vi "State Logic.vi"(0 "TLB' data in":refnum<class "Springboard TLB`.lvclass">, 1 "process state logic enable":bool, 5 "trigger queue in":refnum<queue>, 7 "action queue in":refnum<queue>, 11 "error in":errorcluster) -> (4 "TLB' data out":refnum<class "Springboard TLB`.lvclass">, 15 "error out":errorcluster)   [LabVIEW 2018, in "Springboard TLB`.lvlib" / "Springboard TLB`.lvclass"]
doc: "Control process for TLB' template.\n\n<B>Input Parameters</B>\n\n<B>TLB' data in</B> is the templates' private data.\n\n<B>process state logic enable</B> enable state logic change.\n\n<B>trigger queue in</B> is a reference to a queue. Use the Create Trigger Queue function to obtain a queue reference. \n\n<B>action queue in</B> is a reference to a queue. Use the Create Action Queue function to obtain a queue reference. \n\n<B>timeout (ms)</B> queue timeout.\n\n<B>error in</B> describes error conditions that occur before this node runs. This input provides standard error in functionality.\n\n<B>Output Parameters</B>\n\n<B>TLB' data out</B> is the templates' private data.\n\n<B>error out</B> contains error information. This output provides standard error out functionality."
uses:
  Springboard TLB`.lvclass
  Application Components/Trigger API/System Trigger Element.ctl
  Application Components/Trigger API/System Trigger.ctl
  Core Components/Actions/System Action Element.ctl
  Springboard TLB`.lvclass/Springboard TLB`.ctl
  State.ctl
  Core Components/Error Handler/TLB` Error Handler.lvclass/TLB` Error Handler.ctl
  Core Components/Error Handler/accessors/Get Action Causing Error.vi
  Core Components/Error Handler/accessors/Get Originating State.vi
  Core Components/Error Handler/accessors/Get Destination State.vi
  Core Components/Error Handler/accessors/Get Executed System Actions.vi
  Core Components/Error Handler/accessors/Get Remaing System Actions.vi
  Core Components/Error Handler/Core/actions/support/Error FLUSH-LOG-DIALOG.vi
  Core Components/Error Handler/Core/actions/support/Error FLUSH-DIALOG.vi
  Application Components/Configuration/Springboard Station Configuration.lvclass
  Application Components/Trigger API/Springboard Trigger API.lvlib
  Core Components/Error Handler/TLB` Error Handler.lvclass
  Core Components/Actions/Actions.lvlib
  Springboard TLB`.lvlib
  <vilib>/Utility/config.llb/NI_LVConfig.lvlib
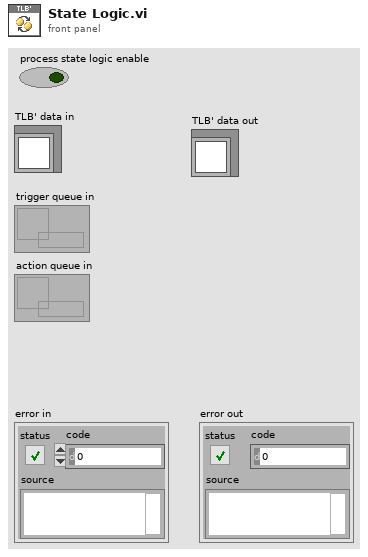
[diagram p1: front panel]
types:
  T1 = typedef "Springboard TLB`.lvlib/Springboard TLB`.lvclass/State.ctl" = enum16{"<Startup>", "Idle", "Evaluate Build Directory", "Creating", "Evaluate Build", "<Shutdown>", "<Error>"}
  T2 = typedef "Springboard TLB`.lvlib/Springboard Trigger API.lvlib/System Trigger.ctl" = enum16{"<None>", "<Return to Safe State Actions>", "<Cache User Parameters>", "<Close Application>", "<Error>", "Create New", "Abort Creation", "Cancel"}
  T3 = typedef "NI_LVConfig.lvlib/Config Data RefNum.ctl" = refnum<k1>
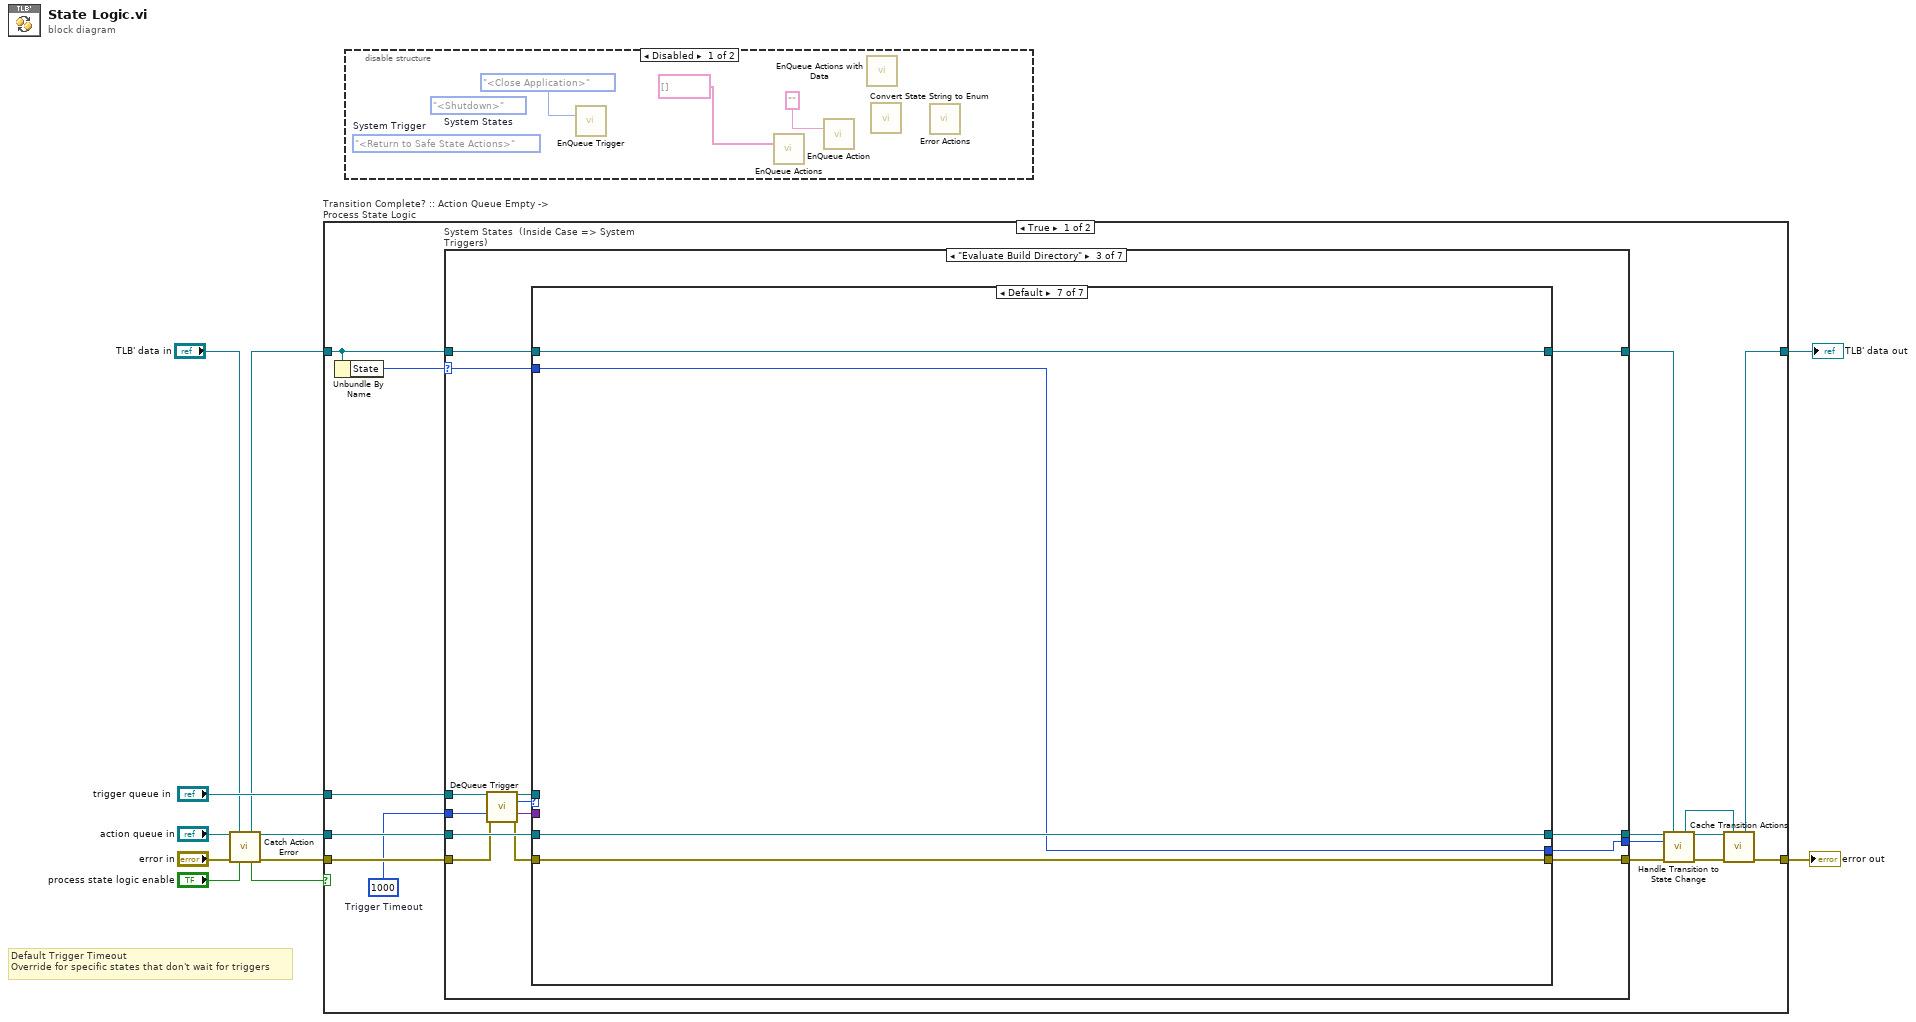
[diagram p0: block diagram]
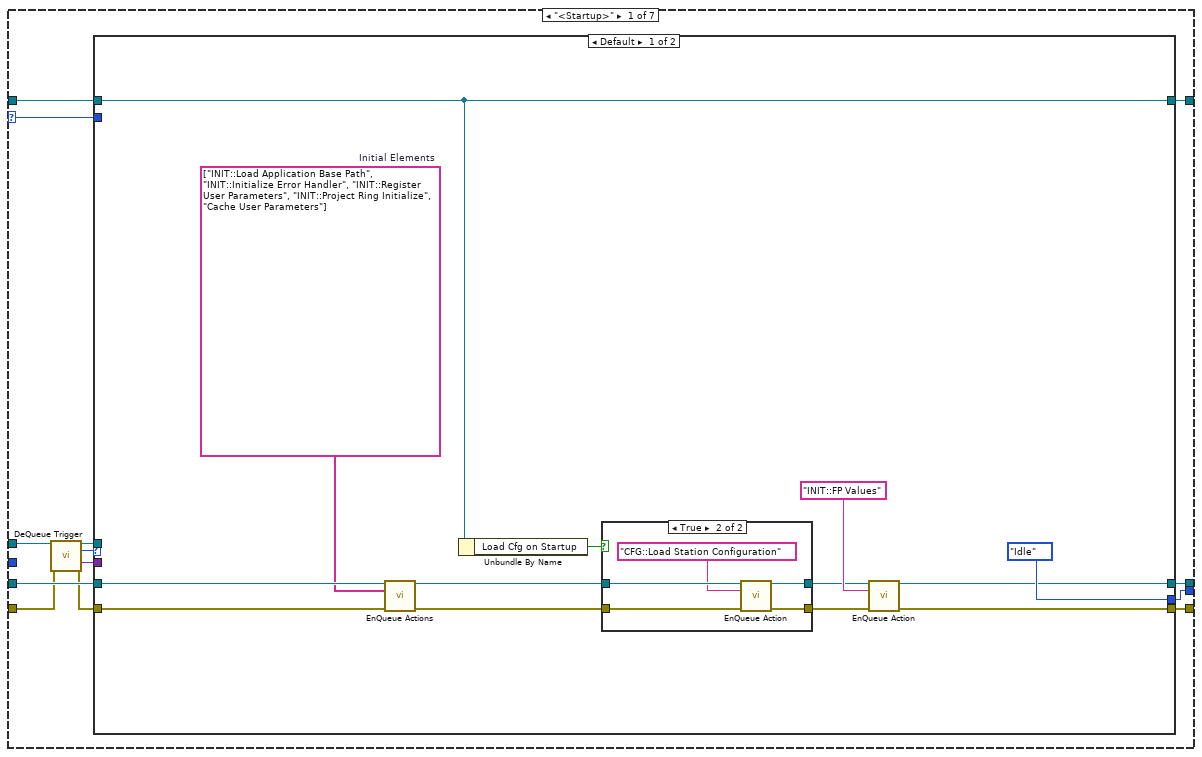
[diagram p3: hidden frame]
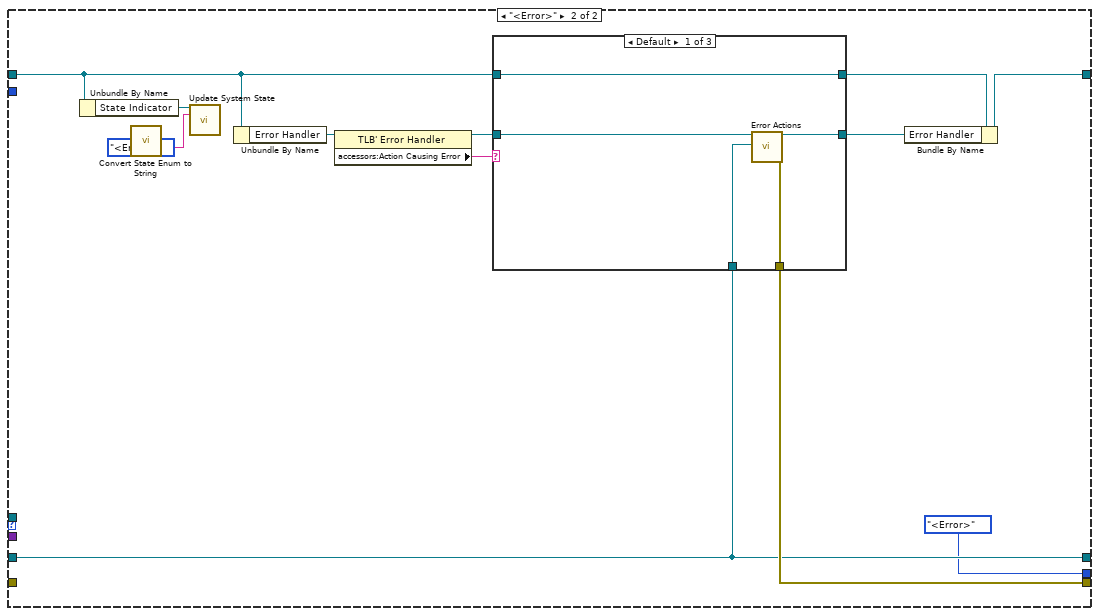
[diagram p5: hidden frame]
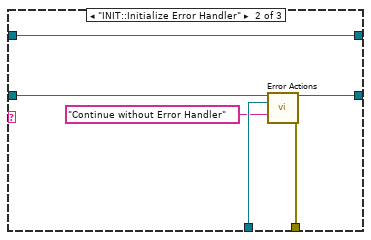
[diagram p6: hidden frame]
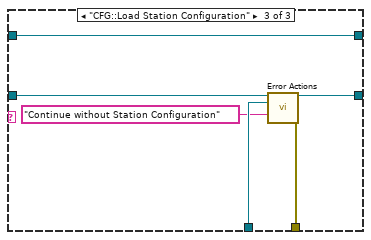
[diagram p7: hidden frame]
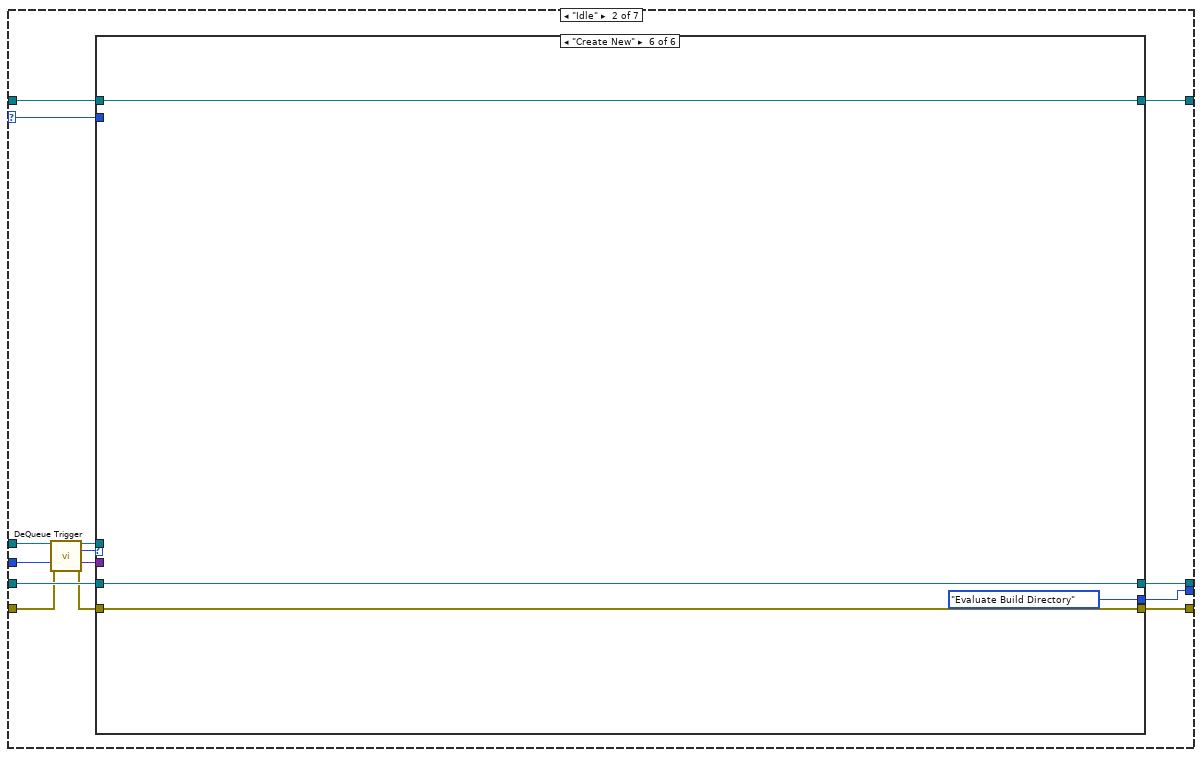
[diagram p8: hidden frame]
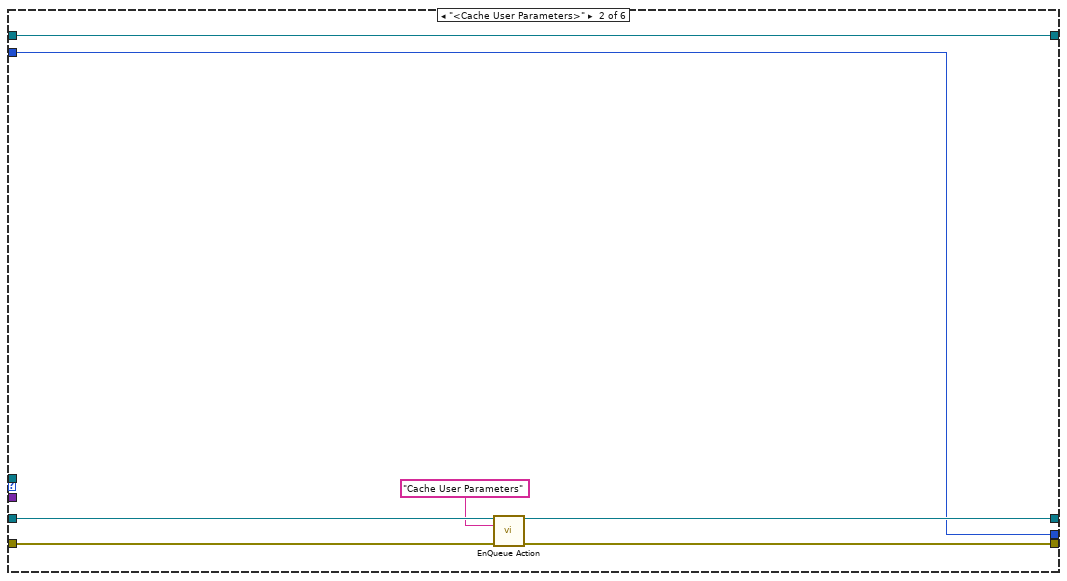
[diagram p10: hidden frame]
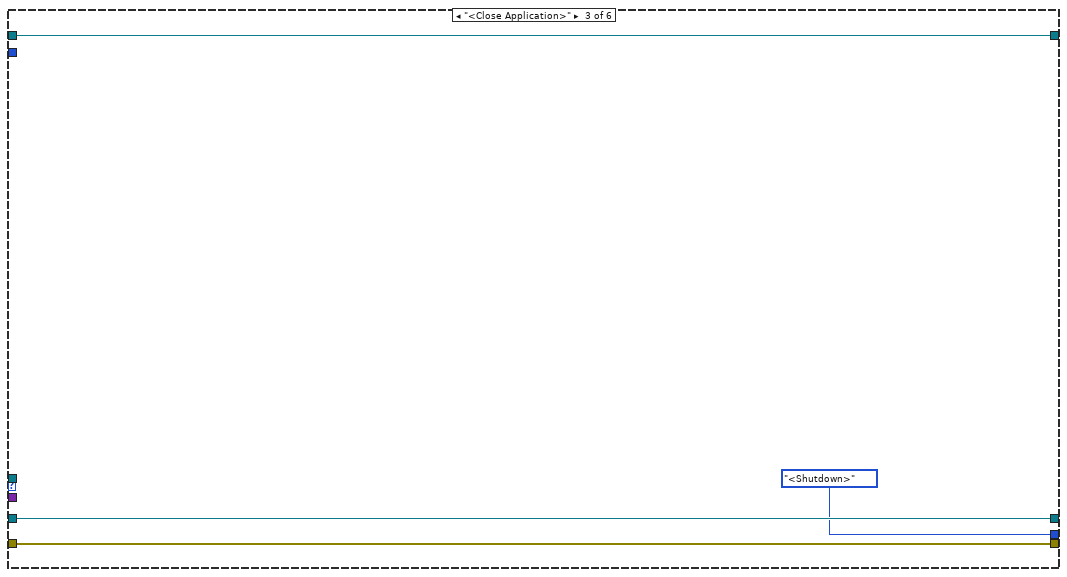
[diagram p11: hidden frame]
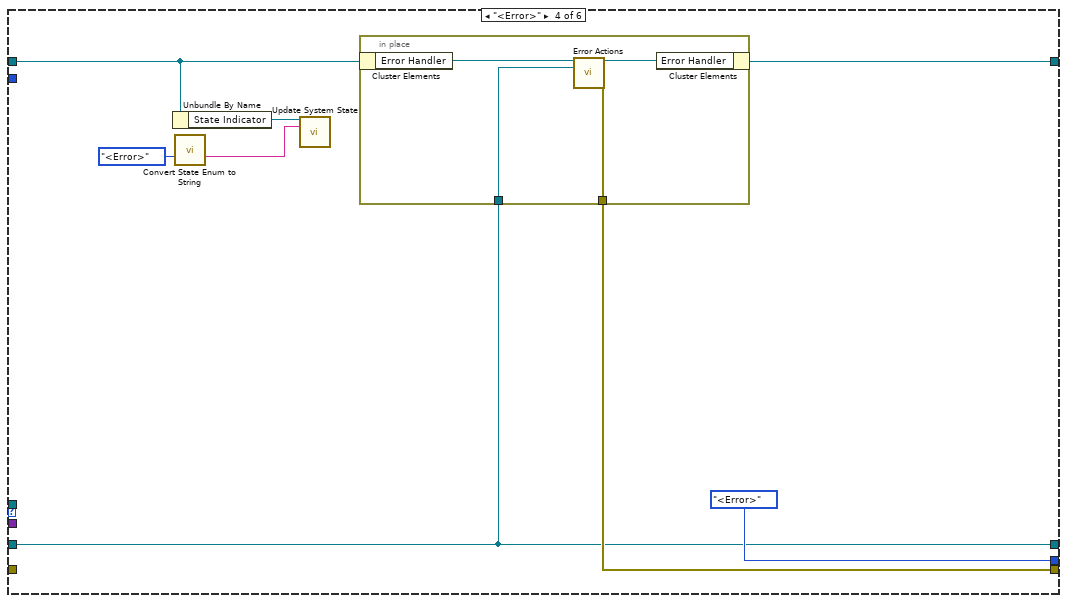
[diagram p12: hidden frame]
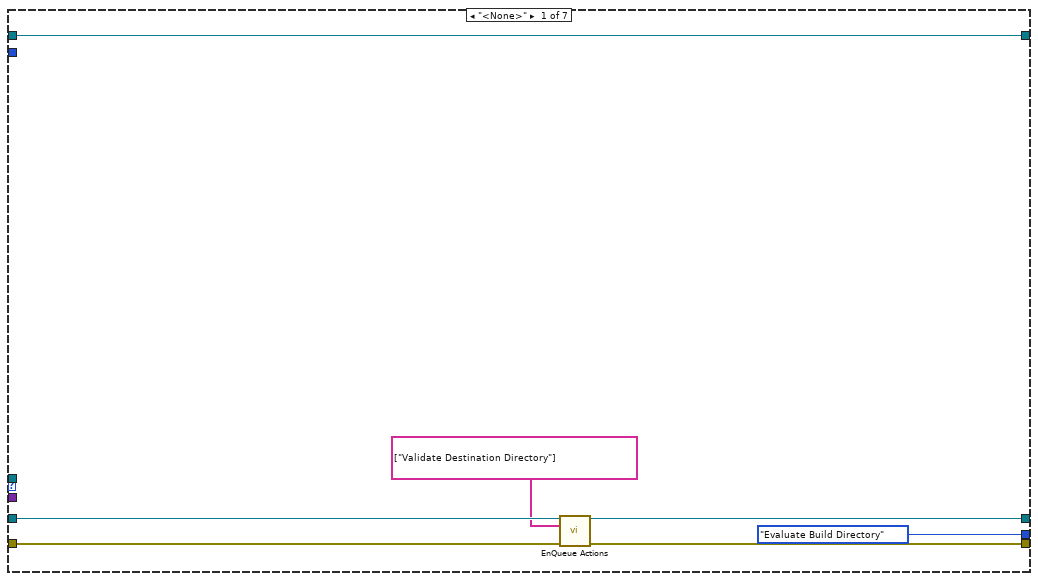
[diagram p14: hidden frame]
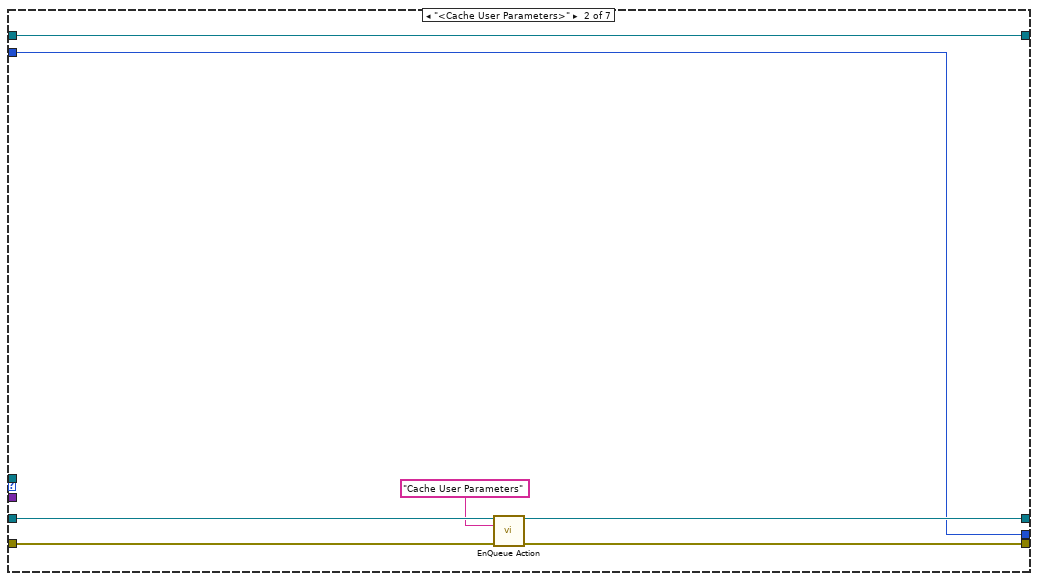
[diagram p15: hidden frame]
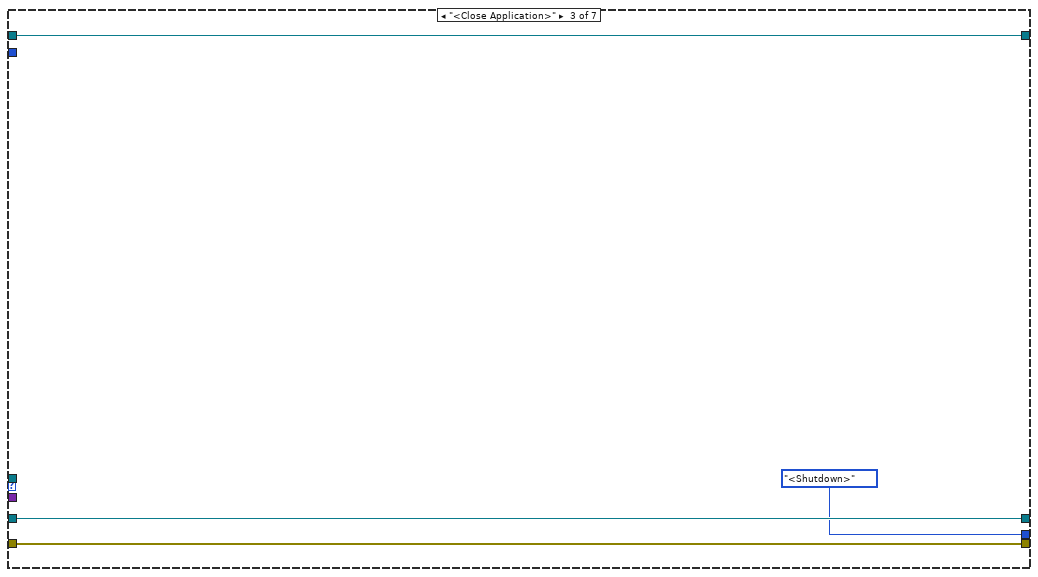
[diagram p16: hidden frame]
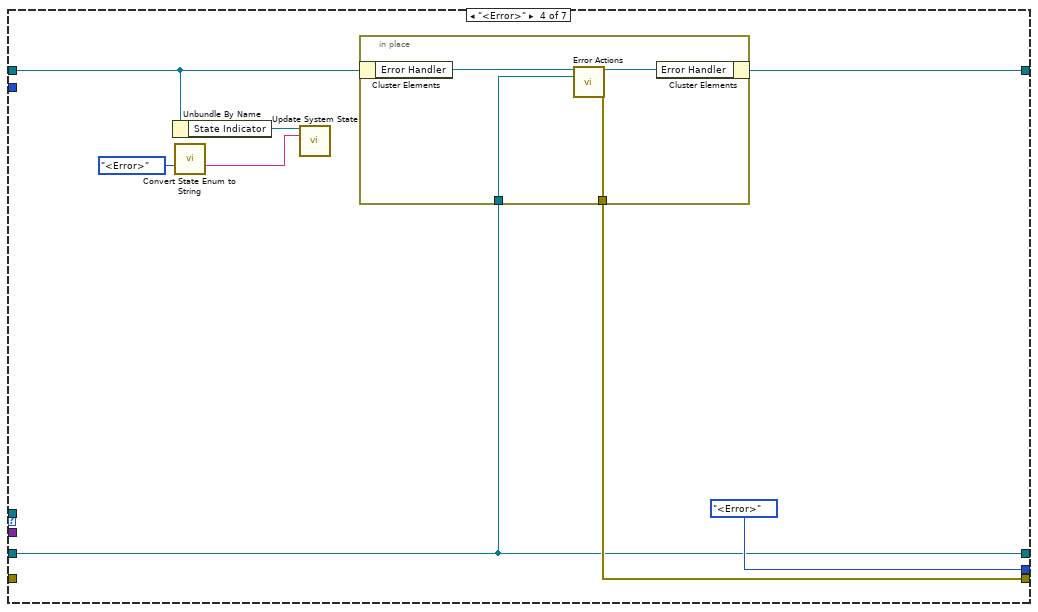
[diagram p17: hidden frame]
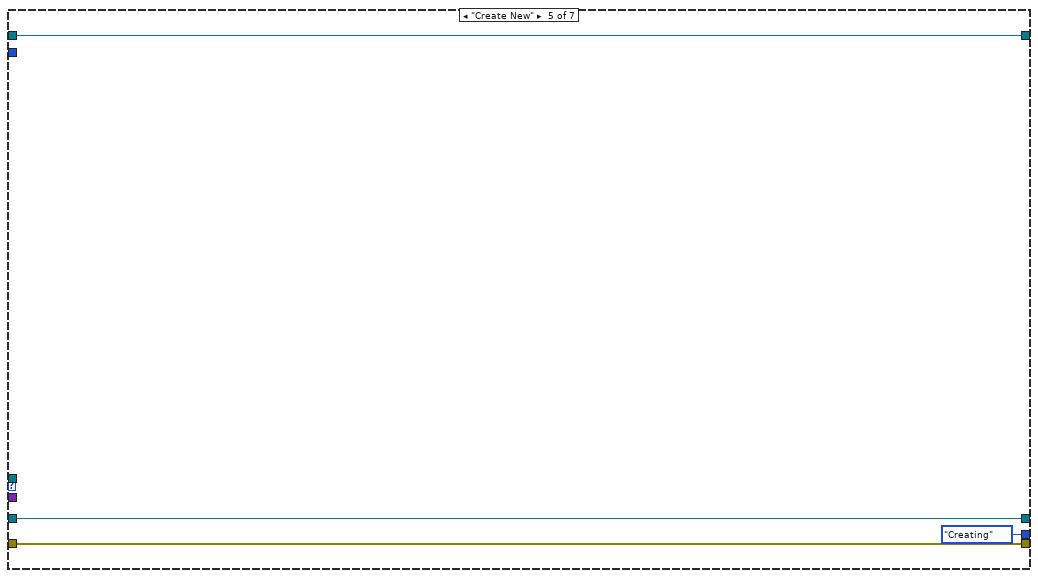
[diagram p18: hidden frame]
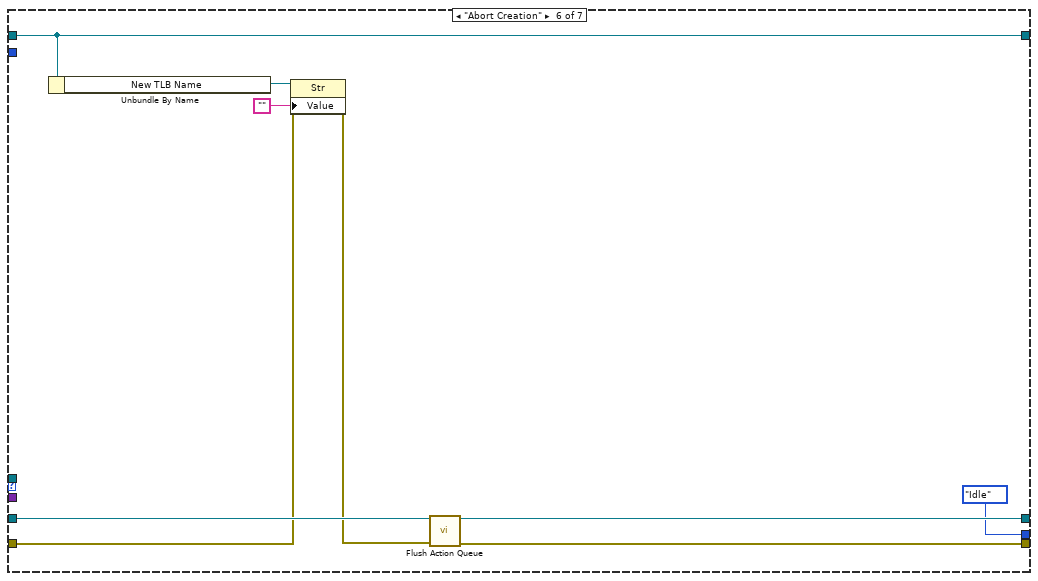
[diagram p19: hidden frame]
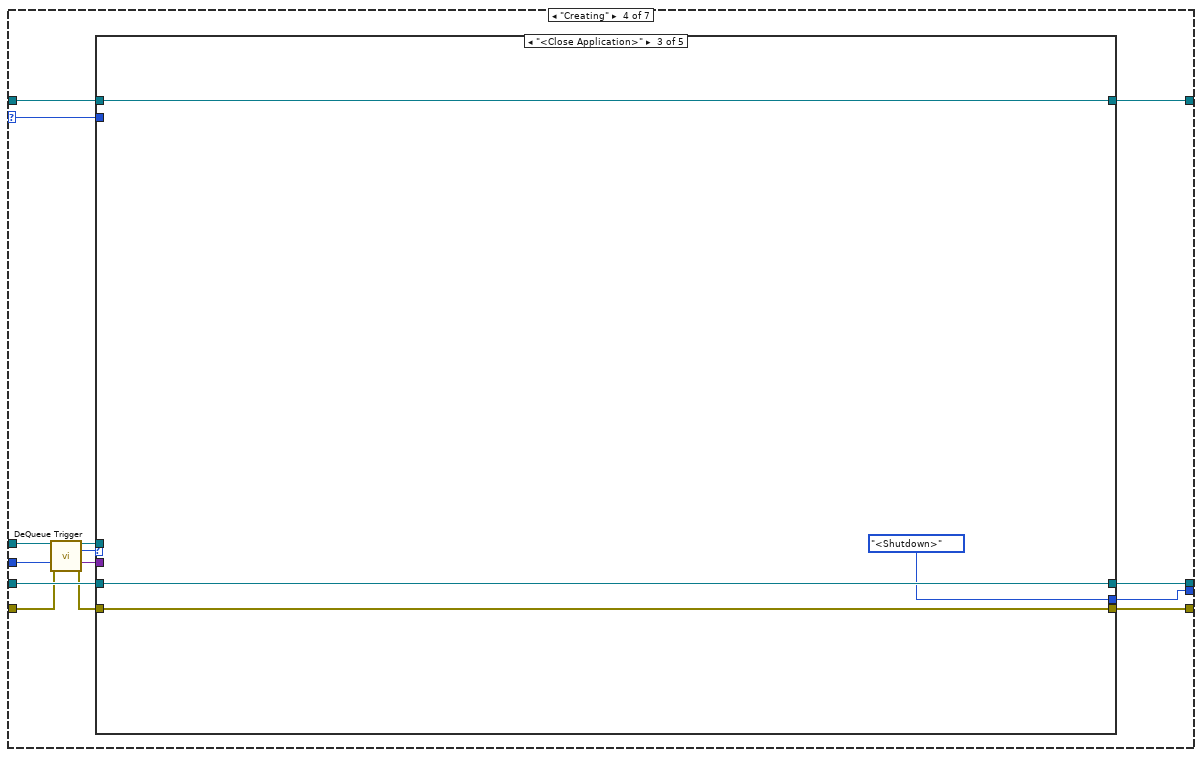
[diagram p20: hidden frame]
diagram:
  # "Default Trigger Timeout\nOverride for specific states that don't wait for triggers"
  n1 = call "Catch Action Error.vi"("action queue in"="action queue in", "TLB' Template in"="TLB' data in", "error in (no error)"="error in", "process state logic enable in"="process state logic enable") -> ("TLB' Template out"=w6:refnum<class "Springboard TLB`.lvclass">, "action queue in"=w2:refnum<queue>, "process state logic enable out"=w4:bool, "error out"=w7:errorcluster)  [unwired: 8 in]
  n2 = case "Transition Complete? :: Action Queue Empty -> Process State Logic" shown="True" w4 {
    tunnel: [w17 w559] -> w10
    tunnel: w6 -> [w22 w559]
    tunnel: w7 -> [w26 w560]
    tunnel: w2 -> [w25 _]
    tunnel: [w20 w560] -> w11
    tunnel: "trigger queue in" -> [w24 _]
    frame True {
      w18 = 1000  # Trigger Timeout
      n3 = Unbundle By Name(w22) -> ("State"=w19:T1)
      n4 = case "System States  (Inside Case => System Triggers)" shown="\"Evaluate Build Directory\"" w19 {
        selector: w19 -> [w27 w92 w141 w202 w250 w324 _]
        tunnel: [w33 w97 w146 w207 w255 w322 w557] -> w15
        tunnel: w22 -> [w34 w98 w147 w208 w256 w323 w557]
        tunnel: w26 -> [w32 w96 w145 w206 w254 w321 w556]
        tunnel: w25 -> [w38 w102 w151 w212 w260 w325 w555]
        tunnel: [w37 w101 w150 w211 w259 w328 w553] -> w23
        tunnel: w24 -> [w39 w103 w152 w213 w261 w329 _]
        tunnel: [w36 w100 w149 w210 w258 w327 w554] -> w16
        tunnel: [w35 w99 w148 w209 w257 w326 State."<Shutdown>" ("State")] -> w12
        tunnel: w18 -> [_ w91 w140 w201 w249 _ _]
        frame "<Startup>" {
          n5 = call "DeQueue Trigger.vi"("trigger queue in"=w39, "error in"=w32) -> ("trigger queue out"=w28:refnum<queue>, "system trigger"=w30:T2, "trigger data"=w29:variant, "error out"=w31:errorcluster)  [unwired: 10 in]
          n6 = case shown="Default" w30 {
            tunnel: w31 -> [w49 _]
            tunnel: w38 -> [w51 w70]
            tunnel: [w40 w71] -> w37
            tunnel: [w42 w70] -> w36
            tunnel: w29 -> [_ _]
            tunnel: [State."Idle" ("State") State."<Error>" ("State")] -> w35
            tunnel: w34 -> [w47 w61]
            tunnel: [w47 w72] -> w33
            tunnel: w28 -> [_ _]
            tunnel: w27 -> [_ _]
            frame Default {
              w50 = string[] ["INIT::Load Application Base Path", "INIT::Initialize Error Handler", "INIT::Register User Parameters", "INIT::Project Ring Initialize", "Cache User Parameters"]  # Initial Elements
              n7 = call "EnQueue Actions.vi"("action queue in"=w51, "actions"=w50, "error in"=w49) -> ("action queue out"=w46:refnum<queue>, "error out"=w48:errorcluster)  [unwired: 11 in]
              n8 = Unbundle By Name(w47) -> ("Load Cfg on Startup"=w45:bool)
              n9 = case shown="True" w45 {
                tunnel: w48 -> [w53 w59]
                tunnel: [w53 w58] -> w41
                tunnel: w46 -> [w54 w57]
                tunnel: [w54 w56] -> w43
                frame False {
                }
                frame True {
                  n10 = call "EnQueue Action.vi"("action queue in"=w57, "action"="CFG::Load Station Configuration", "error in"=w59) -> ("action queue out"=w56:refnum<queue>, "error out"=w58:errorcluster)  [unwired: 11 in]
                }
              }
              n11 = call "EnQueue Action.vi"("action queue in"=w43, "action"="INIT::FP Values", "error in"=w41) -> ("action queue out"=w42:refnum<queue>, "error out"=w40:errorcluster)  [unwired: 11 in]
            }
            frame "<Error>" {
              n12 = Unbundle By Name(w61) -> ("State Indicator"=w65:refnum<user-event>)
              n13 = call "Convert State Enum to String.vi"("state in"=State."<Error>") -> ("state out"=w64:string)  [unwired: 13 in, 1 out]
              n14 = call "Update System State.vi"("State Indicator"=w65, "system state message"=w64) -> ()  [unwired: 13 in, 1 out]
              n15 = Unbundle By Name(w61) -> ("Error Handler"=w67:refnum<class "TLB` Error Handler.lvclass">)
              n16 = property class="TLB' Error Handler"(reference=w67) -> (reference out=w66:refnum<class "TLB` Error Handler.lvclass">, "accessors:Action Causing Error"=w63:string)  [unwired: 1 in, 1 out]
              n17 = case shown="Default" w63 {
                tunnel: [w75 w83 w89] -> w71
                tunnel: w70 -> [w74 w82 w88]
                tunnel: [w76 w81 w87] -> w68
                tunnel: w66 -> [w77 w80 w86]
                tunnel: w61 -> [w73 w78 w84]
                tunnel: [w73 w78 w84] -> w60
                frame Default {
                  n18 = call-poly "Error Actions.vi"("Error Handler in"=w77, "action queue in"=w74) -> ("Error Handler out"=w76:refnum<class "TLB` Error Handler.lvclass">, "error out"=w75:errorcluster)  [unwired: 12 in]
                }
                frame "INIT::Initialize Error Handler" {
                  n19 = call-poly "Error Actions.vi"("Error Handler in"=w80, "action queue in"=w82, "error button text (Return to Safe State)"="Continue without Error Handler") -> ("Error Handler out"=w81:refnum<class "TLB` Error Handler.lvclass">, "error out"=w83:errorcluster)  [unwired: 11 in]
                }
                frame "CFG::Load Station Configuration" {
                  n20 = call-poly "Error Actions.vi"("Error Handler in"=w86, "action queue in"=w88, "error button text (Return to Safe State)"="Continue without Station Configuration") -> ("Error Handler out"=w87:refnum<class "TLB` Error Handler.lvclass">, "error out"=w89:errorcluster)  [unwired: 11 in]
                }
              }
              n21 = Bundle By Name(cluster=w60, "Error Handler"=w68) -> (w72:refnum<class "Springboard TLB`.lvclass">)
            }
          }
        }
        frame "Idle" {
          n22 = call "DeQueue Trigger.vi"("trigger queue in"=w103, "timeout, ms (0)"=w91, "error in"=w96) -> ("trigger queue out"=w90:refnum<queue>, "system trigger"=w94:T2, "trigger data"=w93:variant, "error out"=w95:errorcluster)  [unwired: 9 in]
          n23 = case shown="\"Create New\"" w94 {
            tunnel: w95 -> [w106 w114 w117 _ w133 w137]
            tunnel: w102 -> [w107 w111 w118 w122 w134 w138]
            tunnel: [w106 w112 w117 w124 w133 w137] -> w101
            tunnel: [w107 w110 w118 w122 w134 w138] -> w100
            tunnel: w93 -> [_ _ _ _ _ _]
            tunnel: w98 -> [w105 w113 w116 w121 w132 w136]
            tunnel: [w104 w108 State."<Shutdown>" ("State") State."<Error>" ("State") w131 State."Evaluate Build Directory" ("State")] -> w99
            tunnel: [w105 w113 w116 w123 w132 w136] -> w97
            tunnel: w92 -> [w104 w108 _ _ w131 _]
            tunnel: w90 -> [_ _ _ _ _ _]
            frame "<None>" {
            }
            frame "<Cache User Parameters>" {
              n24 = call "EnQueue Action.vi"("action queue in"=w111, "action"="Cache User Parameters", "error in"=w114) -> ("action queue out"=w110:refnum<queue>, "error out"=w112:errorcluster)  [unwired: 11 in]
            }
            frame "<Close Application>" {
            }
            frame "<Error>" {
              n25 = Unbundle By Name(w121) -> ("State Indicator"=w125:refnum<user-event>)
              n26 = call "Convert State Enum to String.vi"("state in"=State."<Error>") -> ("state out"=w119:string)  [unwired: 13 in, 1 out]
              n27 = call "Update System State.vi"("State Indicator"=w125, "system state message"=w119) -> ()  [unwired: 13 in, 1 out]
              n28 = in-place {
                in-place-border: [w128] -> w124
                in-place-border: w122 -> [w127]
                n29 = in-place-cluster #1(w121) -> ("Error Handler"=w130:refnum<class "TLB` Error Handler.lvclass">)
                n30 = call-poly "Error Actions.vi"("Error Handler in"=w130, "action queue in"=w127) -> ("Error Handler out"=w129:refnum<class "TLB` Error Handler.lvclass">, "error out"=w128:errorcluster)  [unwired: 12 in]
                n31 = in-place-cluster #1("Error Handler"=w129) -> (w123:refnum<class "Springboard TLB`.lvclass">)
              }
            }
            frame Default {
            }
            frame "Create New" {
            }
          }
        }
        frame "Evaluate Build Directory" {
          n32 = call "DeQueue Trigger.vi"("trigger queue in"=w152, "timeout, ms (0)"=w140, "error in"=w145) -> ("trigger queue out"=w139:refnum<queue>, "system trigger"=w143:T2, "trigger data"=w142:variant, "error out"=w144:errorcluster)  [unwired: 9 in]
          n33 = case shown="Default" w143 {
            tunnel: w144 -> [w156 w166 w169 _ w186 w189 w198]
            tunnel: w151 -> [w159 w163 w170 w174 w185 w195 w199]
            tunnel: [w155 w164 w169 w176 w186 w193 w198] -> w150
            tunnel: [w158 w162 w170 w174 w185 w194 w199] -> w149
            tunnel: w142 -> [_ _ _ _ _ _ _]
            tunnel: w147 -> [w154 w165 w168 w173 w184 w191 w197]
            tunnel: [State."Evaluate Build Directory" ("State") w160 State."<Shutdown>" ("State") State."<Error>" ("State") State."Creating" ("State") State."Idle" ("State") w196] -> w148
            tunnel: [w154 w165 w168 w175 w184 w191 w197] -> w146
            tunnel: w141 -> [_ w160 _ _ _ _ w196]
            tunnel: w139 -> [_ _ _ _ _ _ _]
            frame "<None>" {
              n34 = call "EnQueue Actions.vi"("action queue in"=w159, "actions"=string[] ["Validate Destination Directory"], "error in"=w156) -> ("action queue out"=w158:refnum<queue>, "error out"=w155:errorcluster)  [unwired: 11 in]
            }
            frame "<Cache User Parameters>" {
              n35 = call "EnQueue Action.vi"("action queue in"=w163, "action"="Cache User Parameters", "error in"=w166) -> ("action queue out"=w162:refnum<queue>, "error out"=w164:errorcluster)  [unwired: 11 in]
            }
            frame "<Close Application>" {
            }
            frame "<Error>" {
              n36 = Unbundle By Name(w173) -> ("State Indicator"=w177:refnum<user-event>)
              n37 = call "Convert State Enum to String.vi"("state in"=State."<Error>") -> ("state out"=w171:string)  [unwired: 13 in, 1 out]
              n38 = call "Update System State.vi"("State Indicator"=w177, "system state message"=w171) -> ()  [unwired: 13 in, 1 out]
              n39 = in-place {
                in-place-border: [w180] -> w176
                in-place-border: w174 -> [w179]
                n40 = in-place-cluster #2(w173) -> ("Error Handler"=w182:refnum<class "TLB` Error Handler.lvclass">)
                n41 = call-poly "Error Actions.vi"("Error Handler in"=w182, "action queue in"=w179) -> ("Error Handler out"=w181:refnum<class "TLB` Error Handler.lvclass">, "error out"=w180:errorcluster)  [unwired: 12 in]
                n42 = in-place-cluster #2("Error Handler"=w181) -> (w175:refnum<class "Springboard TLB`.lvclass">)
              }
            }
            frame "Create New" {
            }
            frame "Abort Creation" {
              n43 = Unbundle By Name(w191) -> ("New TLB Name"=w190:refnum<vi>)
              n44 = property class="Str"(reference=w190, error in=w189, "Value"="") -> (error out=w188:errorcluster)  [unwired: 1 out]
              n45 = call "Flush Action Queue.vi"("action queue in"=w195, "error in"=w188) -> ("action queue out"=w194:refnum<queue>, "error out"=w193:errorcluster)  [unwired: 11 in, 1 out]
            }
            frame Default {
            }
          }
        }
        frame "Creating" {
          n46 = call "DeQueue Trigger.vi"("trigger queue in"=w213, "timeout, ms (0)"=w201, "error in"=w206) -> ("trigger queue out"=w200:refnum<queue>, "system trigger"=w204:T2, "trigger data"=w203:variant, "error out"=w205:errorcluster)  [unwired: 9 in]
          n47 = case shown="\"<Close Application>\"" w204 {
            tunnel: w205 -> [w217 w227 w230 _ w246]
            tunnel: w212 -> [w220 w224 w231 w235 w247]
            tunnel: [w216 w225 w230 w237 w246] -> w211
            tunnel: [w219 w223 w231 w235 w247] -> w210
            tunnel: w203 -> [_ _ _ _ _]
            tunnel: w208 -> [w215 w226 w229 w234 w245]
            tunnel: [State."Evaluate Build" ("State") w221 State."<Shutdown>" ("State") State."<Error>" ("State") w244] -> w209
            tunnel: [w215 w226 w229 w236 w245] -> w207
            tunnel: w202 -> [_ w221 _ _ w244]
            tunnel: w200 -> [_ _ _ _ _]
            frame "<None>" {
              n48 = call "EnQueue Actions.vi"("action queue in"=w220, "actions"=string[] ["Get Project References", "Open Original Library", "Save Copy Library", "Open Copied Library", "Rename TMPL VIs", "Rename TMPL Libraries"], "error in"=w217) -> ("action queue out"=w219:refnum<queue>, "error out"=w216:errorcluster)  [unwired: 11 in]
            }
            frame "<Cache User Parameters>" {
              n49 = call "EnQueue Action.vi"("action queue in"=w224, "action"="Cache User Parameters", "error in"=w227) -> ("action queue out"=w223:refnum<queue>, "error out"=w225:errorcluster)  [unwired: 11 in]
            }
            frame "<Close Application>" {
            }
            frame "<Error>" {
              n50 = Unbundle By Name(w234) -> ("State Indicator"=w238:refnum<user-event>)
              n51 = call "Convert State Enum to String.vi"("state in"=State."<Error>") -> ("state out"=w232:string)  [unwired: 13 in, 1 out]
              n52 = call "Update System State.vi"("State Indicator"=w238, "system state message"=w232) -> ()  [unwired: 13 in, 1 out]
              n53 = in-place {
                in-place-border: [w241] -> w237
                in-place-border: w235 -> [w240]
                n54 = in-place-cluster #3(w234) -> ("Error Handler"=w243:refnum<class "TLB` Error Handler.lvclass">)
                n55 = call-poly "Error Actions.vi"("Error Handler in"=w243, "action queue in"=w240) -> ("Error Handler out"=w242:refnum<class "TLB` Error Handler.lvclass">, "error out"=w241:errorcluster)  [unwired: 12 in]
                n56 = in-place-cluster #3("Error Handler"=w242) -> (w236:refnum<class "Springboard TLB`.lvclass">)
              }
            }
            frame Default {
            }
          }
        }
        frame "Evaluate Build" {
          n57 = call "DeQueue Trigger.vi"("trigger queue in"=w261, "timeout, ms (0)"=w249, "error in"=w254) -> ("trigger queue out"=w248:refnum<queue>, "system trigger"=w252:T2, "trigger data"=w251:variant, "error out"=w253:errorcluster)  [unwired: 9 in]
          n58 = case shown="\"<Error>\"" w252 {
            tunnel: w253 -> [w263 w296 w299 _ w315]
            tunnel: w260 -> [w268 w293 w300 w304 w316]
            tunnel: [w262 w294 w299 w306 w315] -> w259
            tunnel: [w268 w292 w300 w304 w316] -> w258
            tunnel: w251 -> [_ _ _ _ _]
            tunnel: w256 -> [w266 w295 w298 w303 w314]
            tunnel: [w264 w290 State."<Shutdown>" ("State") State."<Error>" ("State") w313] -> w257
            tunnel: [w265 w295 w298 w305 w314] -> w255
            tunnel: w250 -> [_ w290 _ _ w313]
            tunnel: w248 -> [_ _ _ _ _]
            frame "<None>" {
              n59 = Unbundle By Name(w266) -> ("Build Complete"=w267:bool)
              n60 = case shown="True" w267 {
                tunnel: w266 -> [w271 w275]
                tunnel: [w271 w273] -> w265
                tunnel: [State."Idle" ("State") State."<Shutdown>" ("State")] -> w264
                tunnel: w263 -> [w269 w274]
                tunnel: [w269 w272] -> w262
                frame False {
                }
                frame True {
                  n61 = Unbundle By Name(w275) -> ("Library Path"=w277:refnum<vi>)
                  n62 = Build Array(w277) -> (w276:refnum<vi>[])
                  n63 = in-place {
                    in-place-border: w276 -> [w289]
                    in-place-border: w274 -> [w286]
                    in-place-border: [w279] -> w272
                    n64 = in-place-cluster #4(w275) -> ("Station Configuration"=w288:refnum<class "Springboard Station Configuration.lvclass">)
                    n65 = call-dynamic "Get Cache User Parameters File Path.vi"("error in (no error)"=w286, "Springboard Station Configuration in"=w288) -> ("error out"=w284:errorcluster, "station config INI path"=w285:path, "Springboard Station Configuration out"=w287:refnum<class "Springboard Station Configuration.lvclass">)  [unwired: 7 in]
                    n66 = in-place-cluster #4("Station Configuration"=w287) -> (w273:refnum<class "Springboard TLB`.lvclass">)
                    n67 = call <vilib>:"Open Config Data.vi"("error in (no error)"=w284, "configuration file path"=w285) -> ("error out"=w283:errorcluster, "refnum"=w282:T3)  [unwired: 7 in, 1 out]
                    n68 = call "Write Anything.vi"("refnum"=w282, "user parameter references in"=w289, "error in"=w283) -> ("refnum out"=w281:T3, "error out"=w280:errorcluster)  [unwired: 11 in]
                    n69 = call <vilib>:"Close Config Data.vi"("error in (no error)"=w280, "refnum"=w281) -> ("error out"=w279:errorcluster)  [unwired: 8 in, 1 out]
                  }
                }
              }
            }
            frame "<Cache User Parameters>" {
              n70 = call "EnQueue Action.vi"("action queue in"=w293, "action"="Cache User Parameters", "error in"=w296) -> ("action queue out"=w292:refnum<queue>, "error out"=w294:errorcluster)  [unwired: 11 in]
            }
            frame "<Close Application>" {
            }
            frame "<Error>" {
              n71 = Unbundle By Name(w303) -> ("State Indicator"=w307:refnum<user-event>)
              n72 = call "Convert State Enum to String.vi"("state in"=State."<Error>") -> ("state out"=w301:string)  [unwired: 13 in, 1 out]
              n73 = call "Update System State.vi"("State Indicator"=w307, "system state message"=w301) -> ()  [unwired: 13 in, 1 out]
              n74 = in-place {
                in-place-border: [w310] -> w306
                in-place-border: w304 -> [w309]
                n75 = in-place-cluster #5(w303) -> ("Error Handler"=w312:refnum<class "TLB` Error Handler.lvclass">)
                n76 = call-poly "Error Actions.vi"("Error Handler in"=w312, "action queue in"=w309) -> ("Error Handler out"=w311:refnum<class "TLB` Error Handler.lvclass">, "error out"=w310:errorcluster)  [unwired: 12 in]
                n77 = in-place-cluster #5("Error Handler"=w311) -> (w305:refnum<class "Springboard TLB`.lvclass">)
              }
            }
            frame Default {
            }
          }
        }
        frame "<Error>" {
          n78 = call "DeQueue Trigger.vi"("trigger queue in"=w329, "error in"=w321) -> ("trigger queue out"=w320:refnum<queue>, "system trigger"=w319:T2, "trigger data"=w317:variant, "error out"=w318:errorcluster)  [unwired: 10 in]
          n79 = case shown="\"<Return to Safe State Actions>\"" w319 {
            tunnel: w323 -> [w331 w334 w533 w549]
            tunnel: [w332 w344 w542 w548] -> w328
            tunnel: w318 -> [w332 w346 w543 w548]
            tunnel: w325 -> [w333 w347 w544 w551]
            tunnel: [w333 w345 w539 w551] -> w327
            tunnel: [w330 w343 w541 State."<Shutdown>" ("State")] -> w326
            tunnel: w320 -> [_ _ _ _]
            tunnel: w324 -> [w330 _ _ _]
            tunnel: w317 -> [_ _ _ _]
            tunnel: [w331 w342 w533 w549] -> w322
            frame Default {
            }
            frame "<Return to Safe State Actions>" {
              n80 = Unbundle By Name(w334) -> ("Error Handler"=w341:refnum<class "TLB` Error Handler.lvclass">)
              n81 = property class="TLB' Error Handler"(reference=w341) -> ("accessors:Originating State"=w336:string, "accessors:Action Causing Error"=w340:string, "accessors:Destination State"=w339:string, "accessors:Executed System Actions"=w338:string[], "accessors:Remaing System Actions"=w335:string[])  [unwired: 1 in, 2 out]
              n82 = call "Convert State String to Enum.vi"("state in"=w336) -> ("state out"=w337:T1)  [unwired: 13 in, 1 out]
              n83 = case shown="\"Creating\"" w337 {
                selector: w337 -> [w348 w355 w396 w426 _]
                tunnel: w347 -> [w351 w361 w402 w428 w530]
                tunnel: w346 -> [w349 w362 w403 w427 w529]
                tunnel: [w349 w360 w401 w421 w529] -> w344
                tunnel: [w351 w359 w400 w422 w530] -> w345
                tunnel: [w348 w358 w399 w423 State."<Shutdown>" ("State")] -> w343
                tunnel: w334 -> [w350 w352 w393 w420 w532]
                tunnel: [w350 w353 w394 w424 w532] -> w342
                tunnel: w340 -> [_ w357 w398 w425 _]
                tunnel: w339 -> [_ w354 w395 _ _]
                tunnel: w338 -> [_ _ _ w419 _]
                tunnel: w335 -> [_ w356 w397 _ _]
                frame Default {
                }
                frame "<Startup>" {
                  n84 = case shown="Default" w357 {
                    tunnel: w362 -> [w365 w378 w391]
                    tunnel: w361 -> [w366 w379 w392]
                    tunnel: [w365 w377 w390] -> w360
                    tunnel: [w366 w376 w389] -> w359
                    tunnel: [State."<Shutdown>" ("State") State."Idle" ("state out") State."Idle" ("state out")] -> w358
                    tunnel: w356 -> [_ w375 w388]
                    tunnel: w355 -> [_ w367 w381]
                    tunnel: w354 -> [_ _ _]
                    tunnel: w352 -> [w363 w369 w382]
                    tunnel: [w363 w368 w380] -> w353
                    frame Default {
                    }
                    frame "INIT::Initialize Error Handler" {
                      n85 = Search 1D Array(1D array=w375, element="Change State") -> (index of element=w373:i32)  [unwired: 1 in]
                      n86 = Delete From Array(array=w375, length=1, index=w373) -> (array with subset deleted=w374:string[])  [unwired: 1 out]
                      n87 = call "EnQueue Actions.vi"("action queue in"=w379, "actions"=w374, "error in"=w378) -> ("action queue out"=w376:refnum<queue>, "error out"=w377:errorcluster)  [unwired: 11 in]
                      n88 = Bundle By Name(cluster=w369, "State"=w367) -> (w368:refnum<class "Springboard TLB`.lvclass">)
                    }
                    frame "CFG::Load Station Configuration" {
                      n89 = Search 1D Array(1D array=w388, element="Change State") -> (index of element=w386:i32)  [unwired: 1 in]
                      n90 = Delete From Array(array=w388, length=1, index=w386) -> (array with subset deleted=w387:string[])  [unwired: 1 out]
                      n91 = call "EnQueue Actions.vi"("action queue in"=w392, "actions"=w387, "error in"=w391) -> ("action queue out"=w389:refnum<queue>, "error out"=w390:errorcluster)  [unwired: 11 in]
                      n92 = Bundle By Name(cluster=w382, "State"=w381) -> (w380:refnum<class "Springboard TLB`.lvclass">)
                    }
                  }
                }
                frame "Evaluate Build Directory" {
                  n93 = case shown="\"Validate Destination Directory\"" w398 {
                    tunnel: w403 -> [w406 w411]
                    tunnel: w402 -> [w407 w413]
                    tunnel: [w406 w410] -> w401
                    tunnel: [w407 w409] -> w400
                    tunnel: [State."<Shutdown>" ("State") State."Idle" ("State")] -> w399
                    tunnel: w397 -> [_ w412]
                    tunnel: w396 -> [_ _]
                    tunnel: w395 -> [_ _]
                    tunnel: w393 -> [w404 w417]
                    tunnel: [w404 w417] -> w394
                    frame Default {
                    }
                    frame "Validate Destination Directory" {
                      # "reverse action order"
                      n94 = Reverse 1D Array(array=w412) -> (reversed array=w408:string[])
                      n95 = Array Size(array=w408) -> (size(s)=w415:i32)
                      n96 = Initialize Array("Undo", w415) -> (w414:string[])
                      n97 = call "EnQueue Actions.vi"("action queue in"=w413, "actions"=w408, "data in"=w414, "error in"=w411) -> ("action queue out"=w409:refnum<queue>, "error out"=w410:errorcluster)  [unwired: 10 in]
                    }
                  }
                }
                frame "Creating" {
                  n98 = case shown="\"Open Original Library\"" w425 {
                    tunnel: w427 -> [w431 w434 w444 w459 w474 w489 w504 w519]
                    tunnel: w428 -> [w432 w435 w446 w460 w475 w490 w506 w521]
                    tunnel: [w431 w434 w442 w457 w472 w488 w503 w518] -> w421
                    tunnel: [w432 w435 w445 w458 w473 w487 w505 w520] -> w422
                    tunnel: [State."<Shutdown>" ("State") State."Idle" ("state out") State."Idle" ("state out") State."Idle" ("state out") State."Idle" ("state out") State."Idle" ("state out") State."Idle" ("state out") State."Idle" ("state out")] -> w423
                    tunnel: w426 -> [_ w437 w452 w463 w482 w497 w512 w527]
                    tunnel: [w429 w436 w451 w461 w481 w496 w511 w526] -> w424
                    tunnel: w420 -> [w429 w433 w450 w462 w480 w495 w510 w525]
                    tunnel: w419 -> [_ _ w443 w464 w479 w486 w502 w517]
                    frame Default {
                    }
                    frame "Validate Destination Directory" {
                      n99 = Bundle By Name(cluster=w433, "State"=w437) -> (w436:refnum<class "Springboard TLB`.lvclass">)
                    }
                    frame "Get Project References" {
                      # "reverse action order"
                      n100 = Reverse 1D Array(array=w443) -> (reversed array=w440:string[])
                      n101 = Build Array (concatenate)(w440, "Validate Destination Directory" ("String")) -> (w439:string[])
                      n102 = Array Size(array=w439) -> (size(s)=w448:i32)
                      n103 = Initialize Array("Undo", w448) -> (w447:string[])
                      n104 = call "EnQueue Actions.vi"("action queue in"=w446, "actions"=w439, "data in"=w447, "error in"=w444) -> ("action queue out"=w445:refnum<queue>, "error out"=w442:errorcluster)  [unwired: 10 in]
                      n105 = Bundle By Name(cluster=w450, "State"=w452) -> (w451:refnum<class "Springboard TLB`.lvclass">)
                    }
                    frame "Open Original Library" {
                      # "reverse action order"
                      n106 = Reverse 1D Array(array=w464) -> (reversed array=w455:string[])
                      n107 = Build Array (concatenate)(w455, "Validate Destination Directory" ("String")) -> (w454:string[])
                      n108 = Array Size(array=w454) -> (size(s)=w466:i32)
                      n109 = Initialize Array("Undo", w466) -> (w465:string[])
                      n110 = call "EnQueue Actions.vi"("action queue in"=w460, "actions"=w454, "data in"=w465, "error in"=w459) -> ("action queue out"=w458:refnum<queue>, "error out"=w457:errorcluster)  [unwired: 10 in]
                      n111 = Bundle By Name(cluster=w462, "State"=w463) -> (w461:refnum<class "Springboard TLB`.lvclass">)
                    }
                    frame "Save Copy Library" {
                      # "reverse action order"
                      n112 = Reverse 1D Array(array=w479) -> (reversed array=w470:string[])
                      n113 = Build Array (concatenate)(w470, "Validate Destination Directory" ("String")) -> (w469:string[])
                      n114 = Array Size(array=w469) -> (size(s)=w477:i32)
                      n115 = Initialize Array("Undo", w477) -> (w476:string[])
                      n116 = call "EnQueue Actions.vi"("action queue in"=w475, "actions"=w469, "data in"=w476, "error in"=w474) -> ("action queue out"=w473:refnum<queue>, "error out"=w472:errorcluster)  [unwired: 10 in]
                      n117 = Bundle By Name(cluster=w480, "State"=w482) -> (w481:refnum<class "Springboard TLB`.lvclass">)
                    }
                    frame "Open Copied Library" {
                      # "reverse action order"
                      n118 = Reverse 1D Array(array=w486) -> (reversed array=w493:string[])
                      n119 = Build Array (concatenate)(w493, "Validate Destination Directory" ("String")) -> (w484:string[])
                      n120 = Array Size(array=w484) -> (size(s)=w492:i32)
                      n121 = Initialize Array("Undo", w492) -> (w491:string[])
                      n122 = call "EnQueue Actions.vi"("action queue in"=w490, "actions"=w484, "data in"=w491, "error in"=w489) -> ("action queue out"=w487:refnum<queue>, "error out"=w488:errorcluster)  [unwired: 10 in]
                      n123 = Bundle By Name(cluster=w495, "State"=w497) -> (w496:refnum<class "Springboard TLB`.lvclass">)
                    }
                    frame "Rename TMPL VIs" {
                      # "reverse action order"
                      n124 = Reverse 1D Array(array=w502) -> (reversed array=w500:string[])
                      n125 = Build Array (concatenate)(w500, "Validate Destination Directory" ("String")) -> (w499:string[])
                      n126 = Array Size(array=w499) -> (size(s)=w508:i32)
                      n127 = Initialize Array("Undo", w508) -> (w507:string[])
                      n128 = call "EnQueue Actions.vi"("action queue in"=w506, "actions"=w499, "data in"=w507, "error in"=w504) -> ("action queue out"=w505:refnum<queue>, "error out"=w503:errorcluster)  [unwired: 10 in]
                      n129 = Bundle By Name(cluster=w510, "State"=w512) -> (w511:refnum<class "Springboard TLB`.lvclass">)
                    }
                    frame "Rename TMPL Libraries" {
                      # "backout what you just did... 1, 2, 3 to 3, 2, 1"
                      n130 = Reverse 1D Array(array=w517) -> (reversed array=w515:string[])
                      n131 = Build Array (concatenate)(w515, "Validate Destination Directory" ("String")) -> (w514:string[])
                      n132 = Array Size(array=w514) -> (size(s)=w523:i32)
                      n133 = Initialize Array("Undo", w523) -> (w522:string[])
                      n134 = call "EnQueue Actions.vi"("action queue in"=w521, "actions"=w514, "data in"=w522, "error in"=w519) -> ("action queue out"=w520:refnum<queue>, "error out"=w518:errorcluster)  [unwired: 10 in]
                      n135 = Bundle By Name(cluster=w525, "State"=w527) -> (w526:refnum<class "Springboard TLB`.lvclass">)
                    }
                  }
                }
                frame "<Shutdown>" {
                }
              }
            }
            frame "<Close Application>" {
              n136 = Unbundle By Name(w533) -> ("Error Handler"=w540:refnum<class "TLB` Error Handler.lvclass">)
              n137 = property class="TLB' Error Handler"(reference=w540) -> ("accessors:Originating State"=w538:string, "accessors:Action Causing Error"=w534:string, "accessors:Destination State"=w535:string, "accessors:Executed System Actions"=w536:string[])  [unwired: 1 in, 2 out]
              n138 = call "Convert State String to Enum.vi"("state in"=w538) -> ("state out"=w537:T1)  [unwired: 13 in, 1 out]
              n139 = case shown="Default" w537 {
                tunnel: w544 -> [w546]
                tunnel: w543 -> [w545]
                tunnel: [w545] -> w542
                tunnel: [w546] -> w539
                tunnel: [State."<Shutdown>" ("State")] -> w541
                tunnel: w534 -> [_]
                tunnel: w535 -> [_]
                tunnel: w536 -> [_]
                frame Default {
                }
              }
            }
            frame "<Error>" {
              # "If error errors' that is probably really bad and we should end the program"
            }
          }
        }
        frame "<Shutdown>" {
          n140 = call "EnQueue Actions.vi"("action queue in"=w555, "actions"=string[] ["Exit"], "error in"=w556) -> ("action queue out"=w554:refnum<queue>, "error out"=w553:errorcluster)  [unwired: 11 in]
        }
      }
      n141 = call "Handle Transition to State Change.vi"("action queue in"=w16, "TLB' Template in"=w15, "Destination State"=w12, "error in (no error)"=w23) -> ("TLB' Template out"=w14:refnum<class "Springboard TLB`.lvclass">, "action queue in"=w13:refnum<queue>, "error out"=w21:errorcluster)  [unwired: 9 in]
      n142 = call "Cache Transition Actions.vi"("action queue in"=w13, "TLB' Template in"=w14, "error in (no error)"=w21) -> ("TLB' Template out"=w17:refnum<class "Springboard TLB`.lvclass">, "error out"=w20:errorcluster)  [unwired: 11 in]
    }
    frame False {
    }
  }
  "error out" <- w11
  "TLB' data out" <- w10
  n143 = disable-structure shown="Disabled" {
    frame Disabled {
      (unwired) System_Trigger."<Return to Safe State Actions>"  # System Trigger
      (unwired) State."<Shutdown>"  # System States
      n144 = call "EnQueue Trigger.vi"("system trigger"=System_Trigger."<Close Application>" ("System Trigger")) -> ()  [unwired: 13 in, 2 out]
      n145 = call "EnQueue Actions.vi"("actions"=string[] [] ("message names")) -> ()  [unwired: 13 in, 2 out]
      n146 = call "EnQueue Action.vi"("action"="" ("Message Name")) -> ()  [unwired: 13 in, 2 out]
      n147 = call "EnQueue Actions with Data.vi"() -> ()  [unwired: 14 in, 2 out]
      n148 = call "Convert State String to Enum.vi"() -> ()  [unwired: 14 in, 2 out]
      n149 = call-poly "Error Actions.vi"() -> ()  [unwired: 14 in, 2 out]
    }
    frame Enabled {
    }
  }
